vi "Settings.vi"(8 "Error In":errorcluster, 10 "Data":variant, 11 "Queues":T3) -> ()   [LabVIEW 2017, in "Server.lvlib" / "Dialogs.lvlib"]
uses:
  Dialogs.lvlib
  Message Queue/CommReferences.ctl
  Message Queue/MessageCluster.ctl
  TypeDefs/ServerINI.ctl
  Oracle/OracleData.ctl
  Message Queue/EnqueueMessage(Single).vi
  Message Queue/Message Queue.lvlib
  Server.lvlib
  Oracle/Oracle.lvlib
panel:
  in  "UpdateGlobal?":bool=TRUE
  in  "UpdateINI?":bool=TRUE
  in  "Cancel":bool
  in  "Current INI Data 2":T1={"ClientTimeout (s)"=30, "LogPath"=path "C:/Users/jgoebel/Documents/GitHub/AEDashboard/ServerLib/Data/ServerLog.tdms", "ErrorsToIgnore"=[], "OracleData"={"DBname"="", "User"="", "Password"=""}}
  out "Current INI Data":T1={"ClientTimeout (s)"=30, "LogPath"=path "C:/Users/jgoebel/Documents/GitHub/AEDashboard/ServerLib/Data/ServerLog.tdms", "ErrorsToIgnore"=[], "OracleData"={"DBname"="", "User"="", "Password"=""}}
  in  "Update":bool
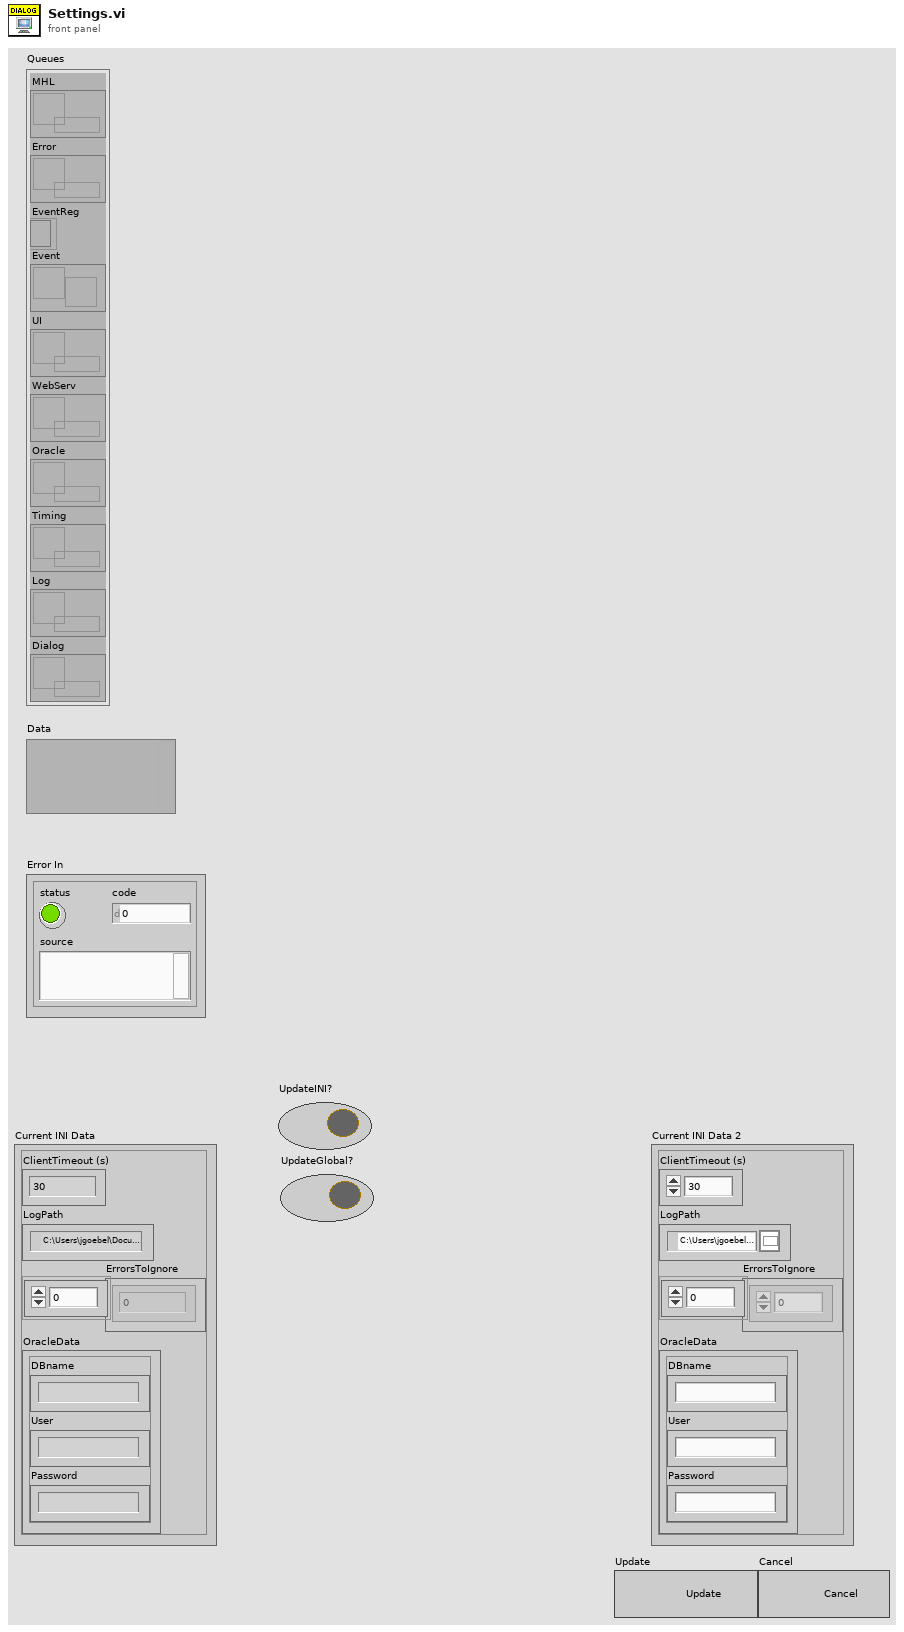
[diagram p1: front panel]
types:
  T1 = typedef "Server.lvlib/ServerINI.ctl" = cluster{"ClientTimeout (s)":u32, "LogPath":path, "ErrorsToIgnore":i32[], "OracleData":T2}
  T2 = typedef "Server.lvlib/Oracle.lvlib/OracleData.ctl" = cluster{"DBname":string, "User":string, "Password":string}
  T3 = typedef "Server.lvlib/Message Queue.lvlib/CommReferences.ctl" = cluster{"MHL":refnum<queue>, "Error":refnum<queue>, "EventReg":refnum<event-registration>, "Event":refnum<user-event>, "UI":refnum<queue>, "WebServ":refnum<queue>, "Oracle":refnum<queue>, "Timing":refnum<queue>, "Log":refnum<queue>, "Dialog":refnum<queue>}
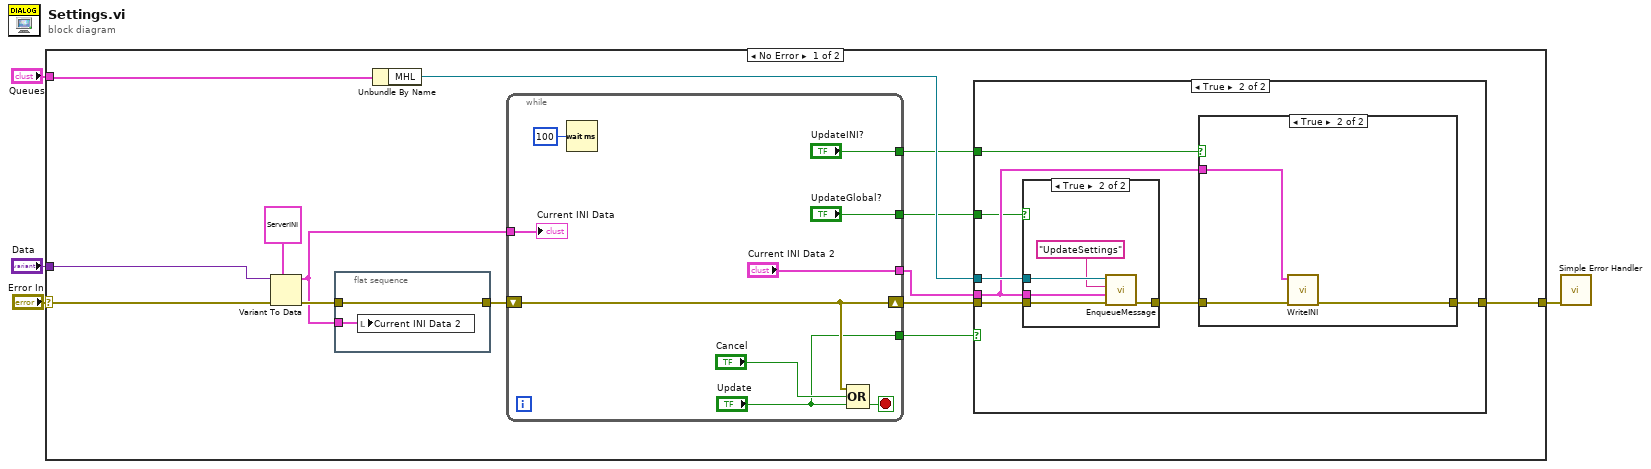
[diagram p0: block diagram]
diagram:
  n1 = case shown="No Error" "Error In" {
    selector: "Error In" -> [w15 w48]
    tunnel: [w9 w48] -> w1
    tunnel: "Queues" -> [w17 _]
    tunnel: "Data" -> [w6 _]
    frame No Error {
      n2 = Variant To Data(error in=w15, type=T1 {"ClientTimeout (s)"=30, "LogPath"=path "C:/Users/jgoebel/Documents/GitHub/AEDashboard/ServerLib/Data/ServerLog.tdms", "ErrorsToIgnore"=[], "OracleData"={"DBname"="", "User"="", "Password"=""}} ("ServerINI"), Variant=w6) -> (data=w5:T1, error out=w8:errorcluster)
      n3 = flat-sequence {
        tunnel: [w20] -> w14
        tunnel: w8 -> [w20]
        tunnel: w5 -> [w19]
        frame #0 {
          n4 = local write "Current INI Data 2"(w19) -> ()
        }
      }
      n5 = Unbundle By Name(w17) -> ("MHL"=w16:refnum<queue>)
      n6 = while {
        shift-right: [w28] -> w18
        shift-left: w14 -> [w28]
        tunnel: ["Current INI Data 2"] -> w12
        tunnel: ["Update"] -> w13
        tunnel: ["UpdateINI?"] -> w11
        tunnel: ["UpdateGlobal?"] -> w10
        tunnel: w5 -> [w21]
        stop <- w29 stop-if-true
        n7 = Wait (ms)(milliseconds to wait=u32 100) -> ()  [unwired: 1 out]
        n8 = Compound Arithmetic op=OR(w28, "Cancel", "Update") -> (w29:bool)
        "Current INI Data" <- w21
      }
      n9 = case shown="True" w13 {
        tunnel: w18 -> [w30 w37]
        tunnel: w16 -> [_ w36]
        tunnel: w12 -> [_ w34]
        tunnel: [w30 w33] -> w9
        tunnel: w11 -> [_ w32]
        tunnel: w10 -> [_ w31]
        frame False {
        }
        frame True {
          n10 = case shown="True" w31 {
            tunnel: w37 -> [w38 w43]
            tunnel: w36 -> [_ w42]
            tunnel: [w38 w40] -> w35
            tunnel: w34 -> [_ w39]
            frame False {
            }
            frame True {
              n11 = call-poly "EnqueueMessage.vi"("error in (no error)"=w43, "Message Data"=w39, "Message"="UpdateSettings", "Message Queue"=w42) -> ("error out"=w40:errorcluster)  [unwired: 6 in, 1 out]
            }
          }
          n12 = case shown="True" w32 {
            tunnel: w35 -> [w44 w47]
            tunnel: w34 -> [_ w45]
            tunnel: [w44 w46] -> w33
            frame False {
            }
            frame True {
              n13 = call "WriteINI.vi"("Error In"=w47, "ServerINI"=w45) -> ("Error Out"=w46:errorcluster)  [unwired: 9 in]
            }
          }
        }
      }
    }
    frame Error {
    }
  }
  n14 = call <vilib>:"Simple Error Handler.vi"("error in (no error)"=w1) -> ()  [unwired: 4 in, 5 out]
